vi "TUNA behavior FWD obstacle avoidance.vi"(1 "Behavior\nVelocity":dbl=20.0, 2 "Activate?":bool=TRUE, 3 "IR Sensors":T1(array[cluster])) -> (0 "Obs Avoid Array":dbl[](array[numeric]))   [LabVIEW 2014]
doc: "This vi uses the values from the Bow sensor to create an Obstacle Avoidance Array."
panel:
  out "Waveform Graph":cluster{dbl, dbl, dbl[]}(graph)
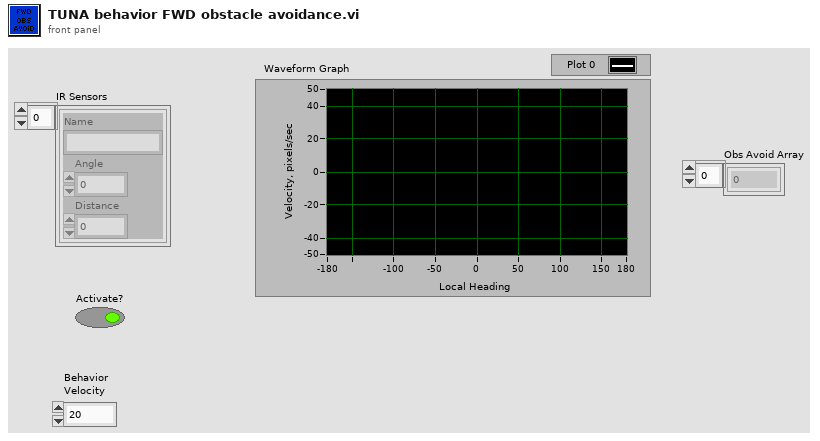
[diagram p1: front panel]
types:
  T1 = cluster{"Name":string, "Angle":dbl, "Distance":dbl}[]
  T2 = cluster{"Name":string, "Angle":dbl, "Distance":dbl}
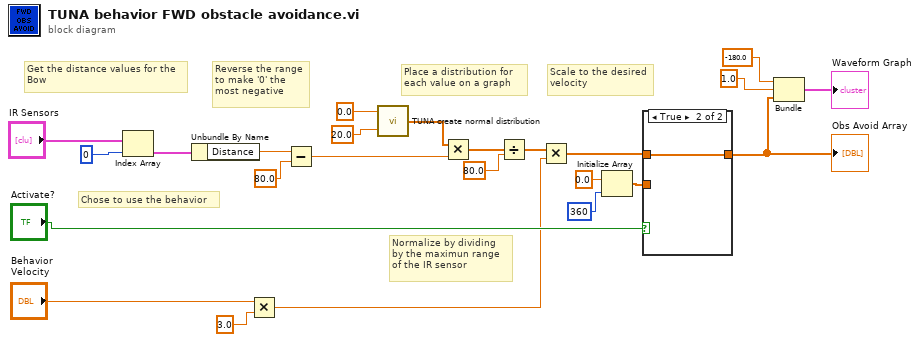
[diagram p0: block diagram]
diagram:
  # "Scale to the desired\nvelocity"
  # "Chose to use the behavior"
  # "Reverse the range\nto make '0' the\nmost negative"
  # "Normalize by dividing\nby the maximun range\nof the IR sensor"
  # "Place a distribution for \neach value on a graph"
  # "Get the distance values for the\nBow"
  n1 = Index Array(array="IR Sensors", index=0) -> (element=w23:T2)
  n2 = Unbundle By Name(w23) -> ("Distance"=w16:dbl)
  n3 = Multiply(x="Behavior\nVelocity", y=3.0) -> (x*y=w3:dbl)
  n4 = Subtract(x=w16, y=80.0) -> (x-y=w14:dbl)
  n5 = call "TUNA create normal distribution.vi"("std (Normal)"=20.0, "mean"=0.0) -> ("ACT array"=w18:dbl[])
  n6 = Multiply(x=w18, y=w14) -> (x*y=w13:dbl[])
  n7 = Divide(x=w13, y=80.0) -> (x/y=w7:dbl[])
  n8 = Multiply(x=w7, y=w3) -> (x*y=w6:dbl[])
  n9 = Initialize Array(0.0 ("element"), 360 ("dimension size")) -> (w9:dbl[])
  n10 = case shown="True" "Activate?" {
    tunnel: w6 -> [_ w26]
    tunnel: w9 -> [w25 _]
    tunnel: [w25 w26] -> w8
    frame False {
    }
    frame True {
    }
  }
  "Obs Avoid Array" <- w8
  n11 = Bundle(-180.0, 1.0, w8) -> (→"Waveform Graph":cluster{dbl, dbl, dbl[]})  [unwired: 1 in]
